vi "Resolve Symbolic Path.vi"(7 "App Inst":refnum<vi>, 8 "error in (no error)":errorcluster, 11 "Path":path=path "<vilib>") -> (0 "error out":errorcluster, 3 "Resolved Path":path)   [LabVIEW 2020, in "Message Rescripter.lvlib"]
uses:
  Message Rescripter.lvlib
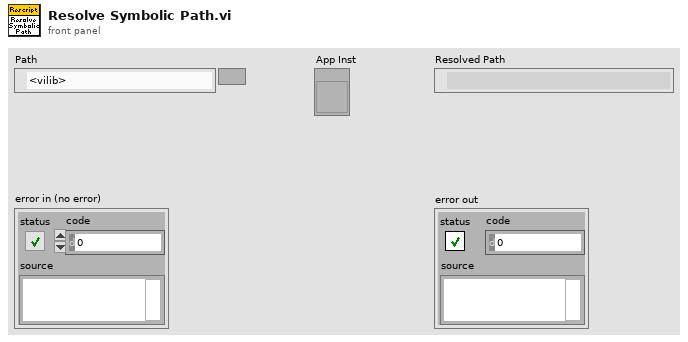
[diagram p1: front panel]
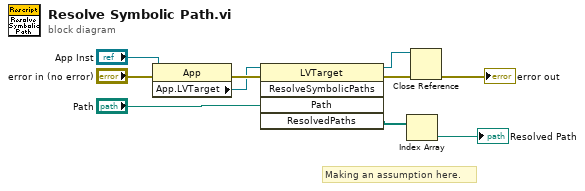
[diagram p0: block diagram]
diagram:
  # "Making an assumption here."
  n1 = property class="App"(reference="App Inst", error in="error in (no error)") -> (error out=w7:errorcluster, "App.LVTarget"=w6:refnum<vi>)  [unwired: 1 out]
  n2 = invoke class="LVTarget" method="ResolveSymbolicPaths"(reference=w6, error in=w7, "Path"="Path") -> (reference out=w4:refnum<vi>, error out=w9:errorcluster, "ResolvedPaths"=w8:path[])  [unwired: 2 in, 2 out]
  n3 = Index Array(array=w8) -> (element=→"Resolved Path":path)  [unwired: 1 in]
  n4 = Close Reference(reference=w4, error in (no error)=w9) -> (error out=→"error out":errorcluster)
